vi "get_mean_speed_from_position.vi"(9 "end":timestamp, 10 "start":timestamp, 11 "lat/lon position":cluster{timestamp[], dbl[], dbl[]} {"?" format="%#_15g"; "?" format="%#_15g"}) -> (1 "dt [s]":dbl, 2 "distance [m]":dbl, 3 "mean speed [m/s]":dbl format="%0.2f")   [LabVIEW 2020]
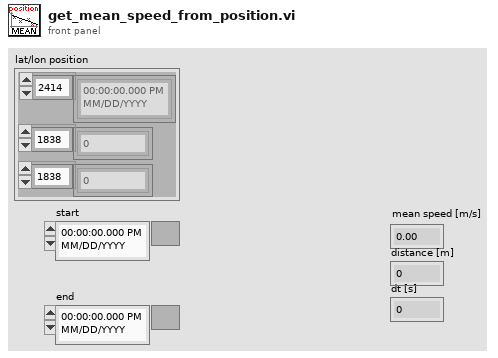
[diagram p1: front panel]
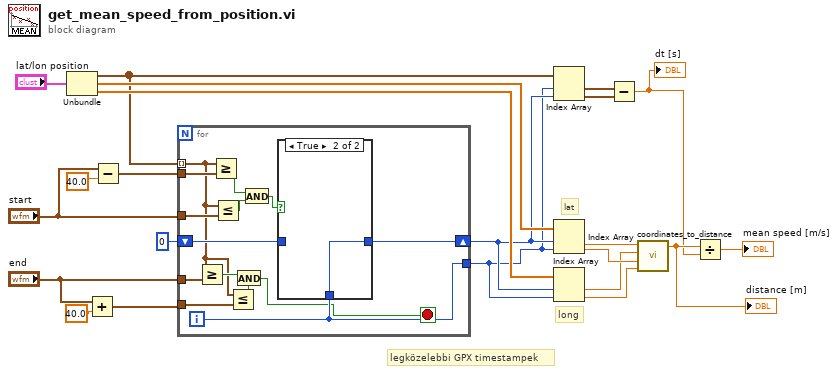
[diagram p0: block diagram]
diagram:
  # "long"
  # "lat"
  # "legközelebbi GPX timestampek"
  n1 = Unbundle("lat/lon position") -> (w9:timestamp[], w15:dbl[], w14:dbl[])
  n2 = Add(x="end", y=40.0) -> (x+y=w17:timestamp)
  n3 = Subtract(x="start", y=40.0) -> (x-y=w20:timestamp)
  n4 = for {
    tunnel: w20 -> [w30]
    tunnel: w9 -> [w23] mode=indexing
    shift-right: [w36] -> w8
    shift-left: 0 -> [w35]
    tunnel: "end" -> [w29]
    tunnel: [w34] -> w7
    tunnel: "start" -> [w25]
    tunnel: w17 -> [w24]
    i -> [w34]
    stop <- w26 stop-if-true
    n5 = Greater Or Equal?(x=w23, y=w29) -> (x >= y?=w28:bool)
    n6 = Greater Or Equal?(x=w23, y=w30) -> (x >= y?=w32:bool)
    n7 = Less Or Equal?(x=w23, y=w25) -> (x <= y?=w31:bool)
    n8 = Less Or Equal?(x=w23, y=w24) -> (x <= y?=w27:bool)
    n9 = And(x=w28, y=w27) -> (x .and. y?=w26:bool)
    n10 = And(x=w32, y=w31) -> (x .and. y?=w33:bool)
    n11 = case shown="True" w33 {
      tunnel: [w37 w38] -> w36
      tunnel: w34 -> [_ w38]
      tunnel: w35 -> [w37 _]
      frame False {
      }
      frame True {
      }
    }
  }
  n12 = Index Array(array=w9, index #1=w7, index #2=w8) -> (element #1=w6:timestamp, element #2=w5:timestamp)
  n13 = Index Array(array=w15, index #1=w8, index #2=w7) -> (element #1=w13:dbl, element #2=w12:dbl)
  n14 = Index Array(array=w14, index #1=w8, index #2=w7) -> (element #1=w11:dbl, element #2=w10:dbl)
  n15 = Subtract(x=w6, y=w5) -> (x-y=w3:dbl)
  "dt [s]" <- w3
  n16 = call "coordinates_to_distance.vi"("end lon"=w10, "end lat"=w12, "start lon"=w11, "start lat"=w13) -> ("distance [m]"=w4:dbl)  [unwired: 7 in]
  "distance [m]" <- w4
  n17 = Divide(x=w4, y=w3) -> (x/y=→"mean speed [m/s]":dbl)
